vi "Enable Measurements.vi"(0 "Register Buses":T1[](array[typedef]), 9 "timeout (s) (10)":dbl=10.0, 11 "error in":errorcluster) -> (4 "Register Buses (out)":T1[](array[typedef]), 15 "error out":errorcluster)   [LabVIEW 2014, in "ni579x Synchronization v2 Host.lvlib"]
doc: "Turn on the measurement circuits on the FPGA. This also involves setting the master, which will be the first FPGA in the array of FPGA VI References."
uses:
  <instrlib>/ni579x/Synchronization/v2/Host/ni579x Synchronization v2 Host.lvlib
  <instrlib>/_niInstr/Register Bus/v0/Host/Public/Register Bus Session.ctl
  <instrlib>/_niInstr/Register Bus/v0/Host/Private/Session Data.ctl
  <instrlib>/ni579x/Synchronization/v2/Shared/ni579x Synchronization Register Addresses.ctl
  <instrlib>/ni579x/Config/v2/Shared/Types/ni579x Register Bus Subsystem ID.ctl
  <instrlib>/_niInstr/Register Bus/v0/Host/Public/Register Write.ctl
  <instrlib>/_niInstr/Register Bus/v0/Host/Public/Register Read Request.ctl
  <vilib>/Utility/error.llb/Error Cluster From Error Code.vi
  <vilib>/ErrorRing/Error Ring.xnode
  <instrlib>/ni579x/Config/v2/Shared/ni579x Config v2 Shared.lvlib
  <instrlib>/_niInstr/Register Bus/v0/Host/niInstr Register Bus v0 Host.lvlib
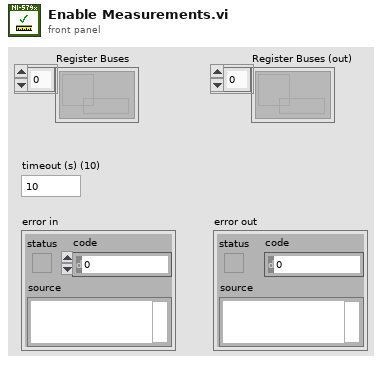
[diagram p1: front panel]
types:
  T1 = typedef "niInstr Register Bus v0 Host.lvlib/Register Bus Session.ctl" = refnum<queue>
  T2 = typedef "niInstr Register Bus v0 Host.lvlib/Register Read Request.ctl" = cluster{"subsystem":u8, "address":u16}
  T3 = typedef "niInstr Register Bus v0 Host.lvlib/Register Write.ctl" = cluster{"subsystem":u8, "address":u16, "data":u32}
  T4 = typedef "ni579x Config v2 Shared.lvlib/ni579x Register Bus Subsystem ID.ctl" = u8
  T5 = typedef "ni579x Synchronization Register Addresses.ctl" = enum16{"Signature", "Current Version", "Oldest Compatible Version", "Scratch Register", "sync.master", "sync.meas.enable", "sync.meas.ready", "sync.meas.arm", "sync.meas.valid", "sync.meas.value", "sync.cptr.adjust", "sync.cptr.period", "sync.meas.oversample factor"}
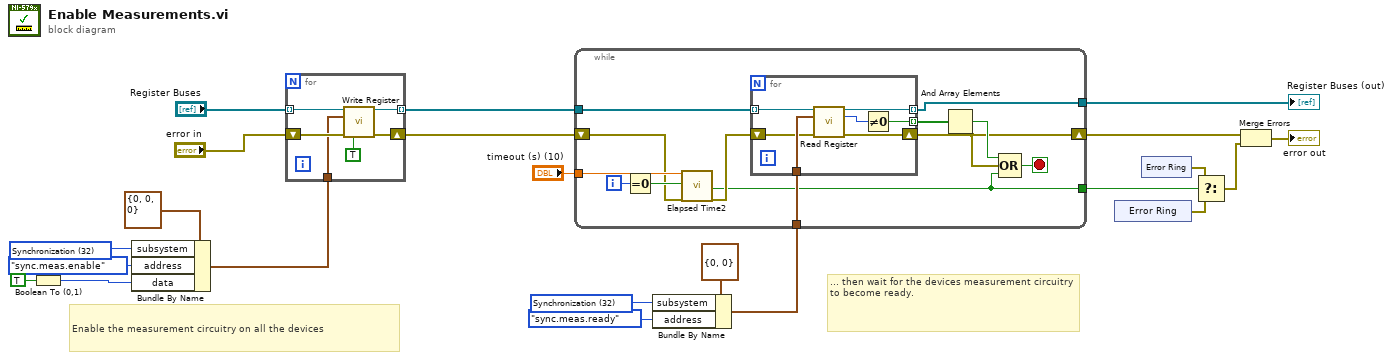
[diagram p0: block diagram]
diagram:
  w11 = T4 32 items=["FAM Register Operation"=0, "User Command"=16, "Synchronization"=32] ("Subsystem ID")
  w16 = T4 32 items=["FAM Register Operation"=0, "User Command"=16, "Synchronization"=32] ("Subsystem ID")
  # "... then wait for the devices measurement circuitry to become ready."
  # "Enable the measurement circuitry on all the devices"
  n1 = Boolean To (0,1)(Boolean=TRUE ("sync.Master")) -> (0, 1=w18:i16)
  n2 = Bundle By Name(cluster=T3 {"subsystem"=0, "address"=0, "data"=0} ("register write"), "subsystem"=w16, "address"=ni579x_Synchronization_Register_Addresses."sync.meas.enable" ("Synchronization Registers"), "data"=w18) -> (w14:T3)
  n3 = for {
    tunnel: "Register Buses" -> [w28] mode=indexing
    tunnel: w14 -> [w26]
    tunnel: [w24] -> w7 mode=indexing
    shift-right: [w23] -> w6
    shift-left: "error in" -> [w27]
    n4 = call <instrlib>:"Write Register.vi"("session in"=w28, "register write"=w26, "error in"=w27, "wait until committed"=TRUE) -> ("session out"=w24:T1, "error out"=w23:errorcluster)  [unwired: 10 in]
  }
  n5 = Bundle By Name(cluster=T2 {"subsystem"=0, "address"=0} ("register read request"), "subsystem"=w11, "address"=ni579x_Synchronization_Register_Addresses."sync.meas.ready" ("Synchronization Registers")) -> (w9:T2)
  n6 = while {
    tunnel: w9 -> [w41]
    tunnel: "timeout (s) (10)" -> [w38]
    tunnel: w7 -> [w36]
    shift-right: [w32] -> w5
    shift-left: w6 -> [w35]
    tunnel: [w30] -> w4
    tunnel: [w29] -> w3
    i -> [w39]
    stop <- w31 stop-if-true
    n7 = Equal To 0?(x=w39) -> (x = 0?=w40:bool)
    n8 = call "Elapsed Time2"("Time Target (s)"=w38, "Reset"=w40, "error in (no error)"=w35) -> ("Time has Elapsed"=w30:bool, "error out"=w37:errorcluster)  [unwired: 9 in, 6 out]
    n9 = for {
      tunnel: w41 -> [w48]
      shift-right: [w45] -> w32
      shift-left: w37 -> [w46]
      tunnel: w36 -> [w44] mode=indexing
      tunnel: [w43] -> w34 mode=indexing
      tunnel: [w42] -> w29 mode=indexing
      n10 = call <instrlib>:"Read Register.vi"("session in"=w44, "register read request"=w48, "error in"=w46) -> ("session out"=w42:T1, "data"=w47:u32, "error out"=w45:errorcluster)  [unwired: 10 in]
      n11 = Not Equal To 0?(x=w47) -> (x != 0?=w43:bool)
    }
    n12 = And Array Elements(Boolean array=w34) -> (logical AND=w33:bool)
    n13 = Compound Arithmetic op=OR(w33, w32, w30) -> (w31:bool)
  }
  "Register Buses (out)" <- w3
  n14 = xnode "Error Ring"() -> ("error out"=w20:errorcluster)
  n15 = xnode "Error Ring"() -> ("error out"=w19:errorcluster)
  n16 = Select(t=w19, s=w4, f=w20) -> (s? t:f=w22:errorcluster)
  n17 = Merge Errors(w5, w22) -> (→"error out":errorcluster)
